vi "SRS_QCM_SubVI  11-10-2017.vi"(0 "VISA Refnum in":refnum<visa-resource-name>, 5 "SRS on?":bool, 11 "error in (no error)":errorcluster) -> (4 "address out":T2, 6 "F,MR output cluster":cluster{"String":string, "String":string}, 8 "freq, MR":T1, 10 "Frequency out":dbl format="%#_8g", 15 "MR out":dbl format="%#_8g")   [LabVIEW 2014]
panel:
  out "error out":errorcluster
  in  "VISA in":refnum<visa-resource-name>="GPIB0::3::INSTR"
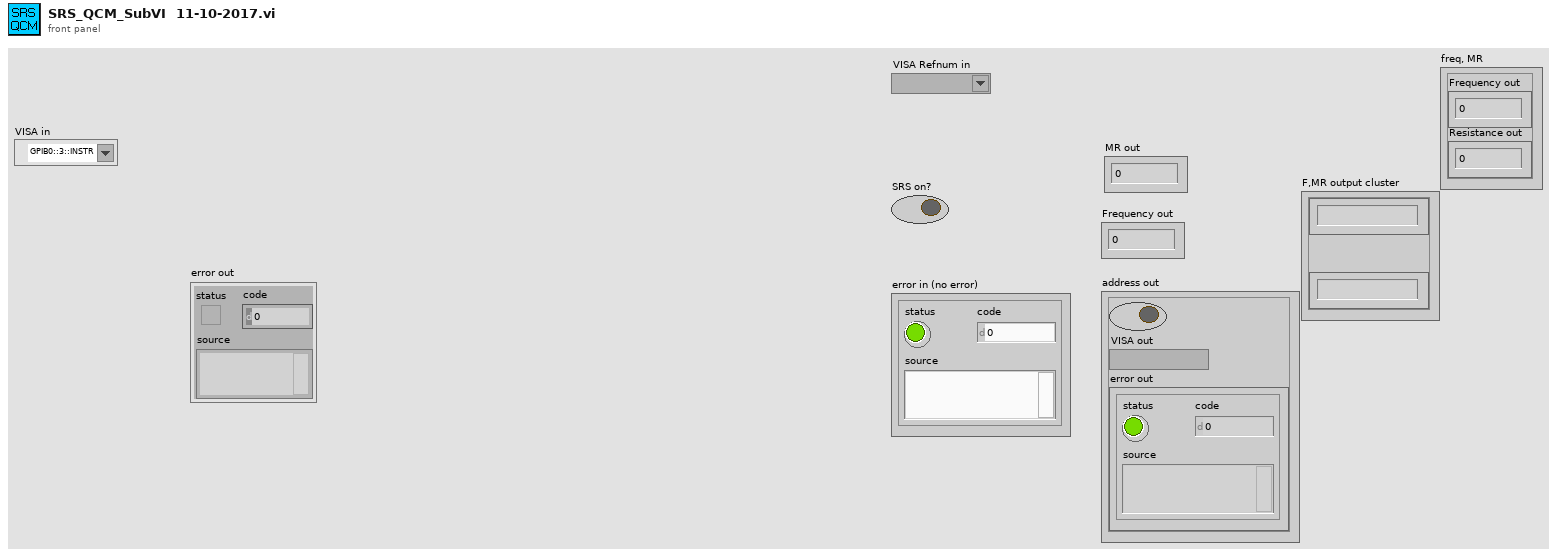
[diagram p1: front panel]
types:
  T1 = cluster{"Frequency out":dbl, "Resistance out":dbl}
  T2 = cluster{"Boolean":bool, "VISA out":refnum<visa-resource-name>, "error out":errorcluster}
  T3 = cluster{"SRS on?":bool, "VISA out":refnum<visa-resource-name>, "error out":errorcluster}
  T4 = cluster{"Frequency out":string, "Resistance out":string}
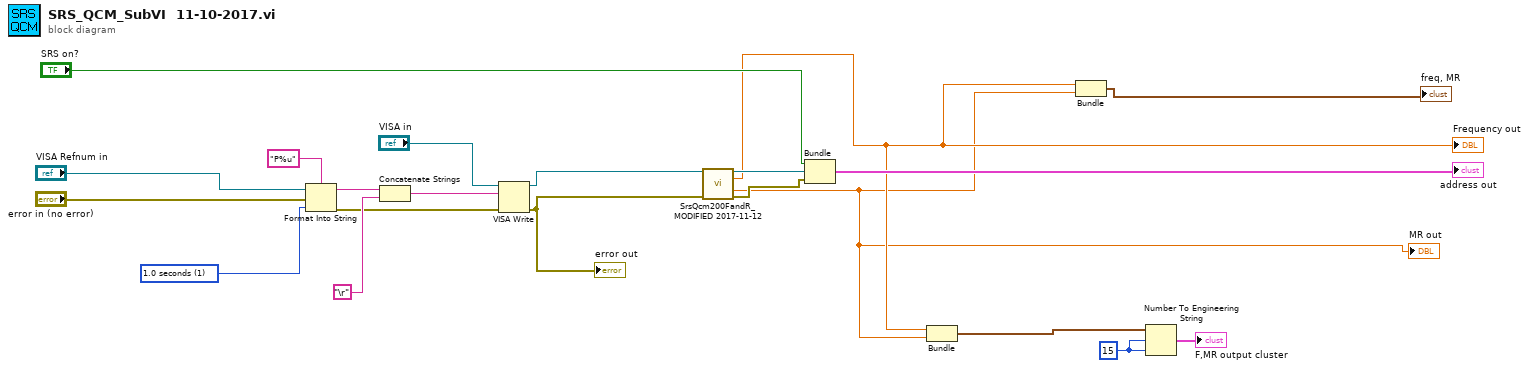
[diagram p0: block diagram]
diagram:
  w7 = u16 1 items=["0.1 seconds", "1.0 seconds", "10.0 seconds"] ("Gate time 2")
  w16 = i16 15 ("width (-)")
  n1 = Format Into String(format string="P%u", initial string="VISA Refnum in", error in="error in (no error)", w7) -> (resulting string=w8:string, error out=w9:errorcluster)
  n2 = Concatenate Strings(w8, "\r") -> (w11:string)
  n3 = VISA Write(VISA resource name="VISA in", write buffer=w11, error in (no error)=w9) -> (VISA resource name out=w3:refnum<visa-resource-name>, error out=w4:errorcluster)  [unwired: 1 out]
  "error out" <- w4
  n4 = call "SrsQcm200FandR_MODIFIED 2017-11-12.vi"("VISA in"=w3, "error in (no error)"=w4) -> ("VISA out"=w21:refnum<visa-resource-name>, "Frequency out"=w15:dbl, "Resistance out"=w1:dbl, "error out"=w20:errorcluster)  [unwired: 10 in]
  "Frequency out" <- w15
  "MR out" <- w1
  n5 = Bundle("SRS on?"="SRS on?", "VISA out"=w21, "error out"=w20) -> (→"address out":T3)  [unwired: 1 in]
  n6 = Bundle("Frequency out"=w15, "Resistance out"=w1) -> (w17:T1)  [unwired: 1 in]
  n7 = Bundle("Frequency out"=w15, "Resistance out"=w1) -> (→"freq, MR":T1)  [unwired: 1 in]
  n8 = Number To Engineering String(2:w16, 3:w16, 4:w17) -> (0:→"F,MR output cluster":T4)  [unwired: 1 in]
